vi "All RUNs Completed.vi"(8 "error in (no error)":errorcluster, 11 "Monkey in":refnum<class "Monkey.lvclass">) -> (0 "error out":errorcluster, 2 "Monkey Status":T1=enum."Ongoing", 3 "Monkey out":refnum<class "Monkey.lvclass">)   [LabVIEW 2020, in "Monkey.lvlib" / "Monkey.lvclass"]
doc: "Clear Current RUN. Pop-up message saying the RUNs are completed. Change global RUN led status"
uses:
  Monkey.lvclass
  C:/Users/marco/Documents/GitHub_Lab/TALOS/talos/Father of all uServices/Father of all uServices/Father of all uServices.lvclass
  Run Utilities/TypeDefs/Monkey Status.ctl
  Monkey Consumer Case Selector.ctl
  Father of all uServices/Father of all uServices Messages/Consumer Msg/Consumer Msg.lvclass/Consumer Msg.ctl
  Ancestor/Ancestor/Ancestor.lvclass/Ancestor.ctl
  Father of all uServices/Father of all uServices/Father of all uServices.lvclass/Father of all uServices.ctl
  Father of all uServices/Father of all uServices Messages/Consumer Msg/Send Consumer.vi
  Support VIs/Substitute Error.vi
  Support VIs/Generate Error.vi
  FGV/Error Memory/Get Error Description.vi
  Support VIs/Get PC name.vi
  Ancestor/Ancestor/Read ID.vi
  Support VIs/Get Class Name.vi
  <vilib>/Utility/error.llb/Clear Errors.vi
  FGV/Error Memory/Error Memory Core.vi
  <vilib>/AdvancedString/Delimited String to 1D String Array.vi
  Support VIs/Circus Root Path.vi
  FGV/Error Memory/Error Crt Lvl checker.vi
  FGV/Error Memory/Error Memory Core.vi/40c8088d-b597-4017-91af-faa98e00292e.vi
  FGV/Error Memory/Error Memory Core.vi/d4a3ab98-063c-4e44-b43d-fbdcfe6c2be2.vi
  Father of all uServices/Father of all uServices/Father of all uServices.lvclass
  C:/Users/marco/Documents/GitHub_Lab/TALOS/builds/Actor Framework PPL/Actor Framework.lvlibp/1abvi3w/vi.lib/ActorFramework/Actor/Actor.lvclass
  builds/Actor Framework PPL/Actor Framework.lvlibp/1abvi3w/vi.lib/ActorFramework/Actor/Read Self Enqueuer.vi
  <userlib>/_OpenG.lib/lvdata/lvdata.llb/Get Strings from Enum__ogtk.vi
  builds/Actor Framework PPL/Actor Framework.lvlibp/1abvi3w/vi.lib/ActorFramework/Message Enqueuer/Enqueue.vi
  Support VIs/Global Memory.vi
  <vilib>/Utility/LVClass/Get LV Class Name.vi
  Support VIs/Is in Packed Library.vi
  Support VIs/TALOS Root path.vi
  Support VIs/Read CSV worksheet.vi
  Support VIs/Global Constants.vi
  <vilib>/Utility/error.llb/General Error Handler.vi
  Support VIs/Error Log.vi
  Father of all uServices/Father of all uServices Messages/Consumer Msg/Consumer Msg.lvclass
  Ancestor/Ancestor/Ancestor.lvclass
  <vilib>/Comparison/Equal/Equal Functor/Equal Functor.lvclass
  Run Utilities/Run Utilities.lvlib
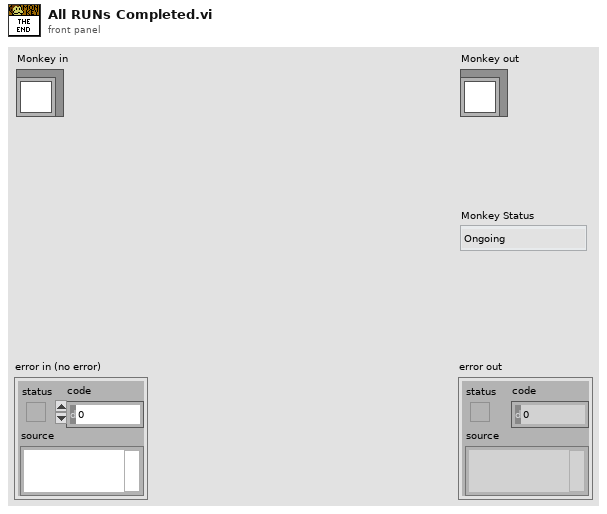
[diagram p1: front panel]
types:
  T1 = typedef "TALOS.lvlib/Run Utilities.lvlib/Monkey Status.ctl" = enum16{"Init", "Paused", "Ongoing", "Stopped", "Finished (no errors)", "Finished (with errors)"}
  T2 = typedef "Monkey.lvlib/Monkey.lvclass/Monkey Consumer Case Selector.ctl" = enum16{"Init", "Update GUI", "New schedule", "Check Script", "Submit Script", "Banana arrived", "Optimiser - evaluate RUN", "Optimiser - update RUN", "Quality Check", "What to do next", "Update Crit Lvl", "Skip Run", "Stop Schedule", "Skip schedule"}
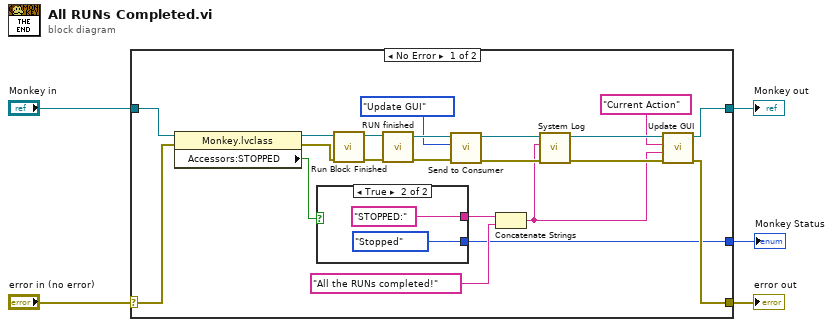
[diagram p0: block diagram]
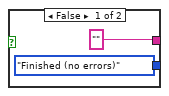
[diagram p2: hidden frame]
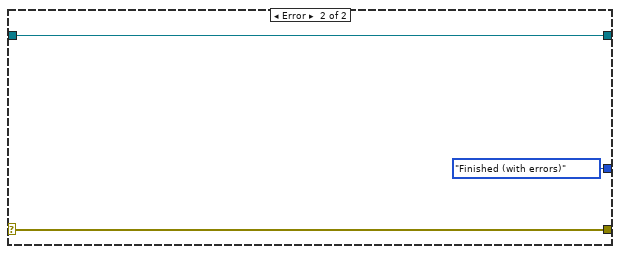
[diagram p3: hidden frame]
diagram:
  n1 = case shown="No Error" "error in (no error)" {
    selector: "error in (no error)" -> [w11 w33]
    tunnel: [w18 w33] -> w4
    tunnel: [w19 w32] -> w2
    tunnel: "Monkey in" -> [w12 w32]
    tunnel: [w16 Monkey_Status."Finished (with errors)" ("Monkey Status")] -> w1
    frame No Error {
      n2 = property class="Monkey.lvclass"(reference=w12, error in=w11) -> (reference out=w10:refnum<class "Monkey.lvclass">, error out=w9:errorcluster, "Accessors:STOPPED"=w14:bool)
      n3 = case shown="True" w14 {
        tunnel: ["" "STOPPED:" ("t")] -> w17
        tunnel: [Monkey_Status."Finished (no errors)" ("Monkey Status") Monkey_Status."Stopped" ("Monkey Status")] -> w16
        frame False {
        }
        frame True {
        }
      }
      n4 = call-dynamic "Run Block Finished.vi"("error in (no error)"=w9, "Monkey in"=w10) -> ("error out"=w7:errorcluster, "Monkey out"=w8:refnum<class "Monkey.lvclass">)  [unwired: 8 in]
      n5 = call-dynamic "RUN finished.vi"("error in (no error)"=w7, "Monkey in"=w8) -> ("error out"=w20:errorcluster, "Monkey out"=w13:refnum<class "Monkey.lvclass">)  [unwired: 8 in]
      n6 = call "Send to Consumer.vi"("error in (no error)"=w20, "Case ID"=Monkey_Consumer_Case_Selector."Update GUI" ("Consumer Case Selector"), "uService Template in"=w13) -> ("error out"=w22:errorcluster, "uService Template out"=w23:refnum<class "Monkey.lvclass">)  [unwired: 7 in]
      n7 = Concatenate Strings(w17, "All the RUNs completed!" ("Text to log")) -> (w15:string)
      n8 = call "System Log.vi"("error in (no error)"=w22, "Text to log"=w15, "uService Template in"=w23) -> ("error out"=w24:errorcluster, "uService Template out"=w26:refnum<class "Monkey.lvclass">)  [unwired: 7 in]
      n9 = call "Update GUI.vi"("error in (no error)"=w24, "Data"=w15, "GUI Item Name"="Current Action", "uService Template in"=w26) -> ("error out"=w18:errorcluster, "uService Template out"=w19:refnum<class "Monkey.lvclass">)  [unwired: 6 in]
    }
    frame Error {
    }
  }
  "error out" <- w4
  "Monkey out" <- w2
  "Monkey Status" <- w1
